vi "TestPage2.vi"() -> ()   [LabVIEW 2013]
panel:
  in  "MainPage":bool
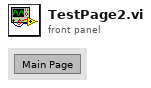
[diagram p1: front panel]
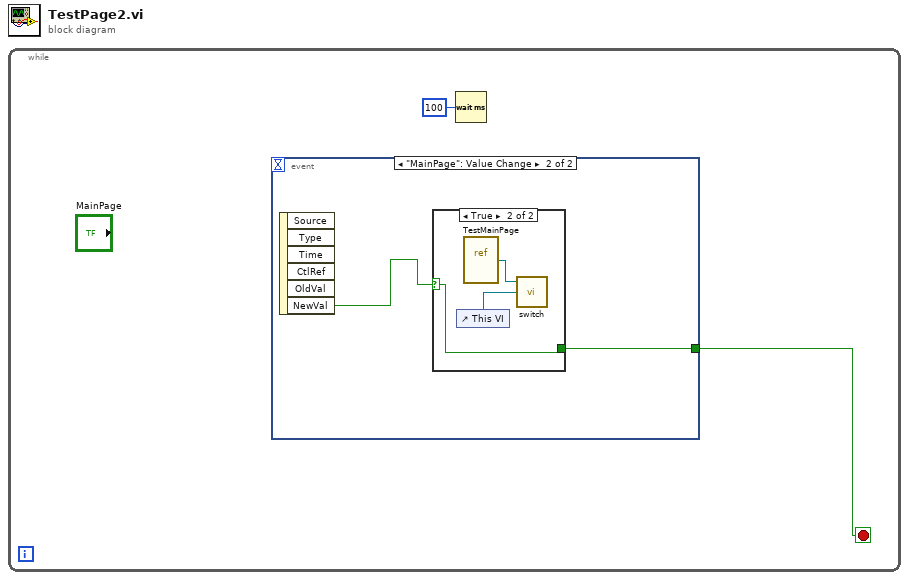
[diagram p0: block diagram]
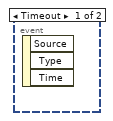
[diagram p2: hidden frame]
diagram:
  n1 = while {
    stop <- w1 stop-if-true
    n2 = event shown="[1] \"MainPage\": Value Change" {
      selector: _ -> [_ _]
      dyn-events: _ -> [_ _]
      timeout: _ -> [_ _]
      tunnel: [_ w3] -> w1
      event Timeout {
        n3 = event-data() -> ()  [unwired: 1 in, 3 out]
      }
      event "MainPage": Value Change {
        n4 = event-data() -> ("NewVal"=w4:bool)  [unwired: 1 in, 5 out]
        n5 = case shown="True" w4 {
          selector: w4 -> [_ w5]
          tunnel: [_ w5] -> w3
          frame False {
          }
          frame True {
            n6 = control-ref of="This VI"() -> (w6:refnum<vi>)
            n7 = vi-ref "TestMainPage.vi"() -> (w7:refnum<vi>)
            n8 = call "switch.vi"("vi close"=w6, "vi open"=w7) -> ()  [unwired: 1 in, 1 out]
          }
        }
      }
    }
    n9 = Wait (ms)(milliseconds to wait=u32 100) -> ()  [unwired: 1 out]
  }
